vi "_uintGetUintBase.vi"(8 "Error in (no error)":errorcluster, 11 "UintClass in":refnum<class "UintClass.lvclass">) -> (0 "Error out":errorcluster, 1 "Base out":T1=10 caption="Base (decimal)" items=["Binary"=2, "Octal"=8, "Decimal"=10, "Hexadecimal"=16, "Hexatrigesimal"=36, "ASCII"=64], 2 "Uint out":u8[](array[numeric]), 3 "UintClass out":refnum<class "UintClass.lvclass">)   [LabVIEW 2011]
uses:
  UintClass.lvclass
  enumBase.ctl
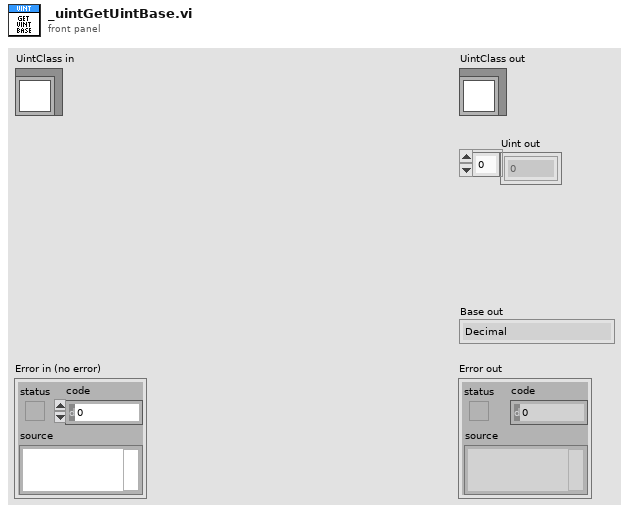
[diagram p1: front panel]
types:
  T1 = typedef "UintClass.lvclass/enumBase.ctl" = u16
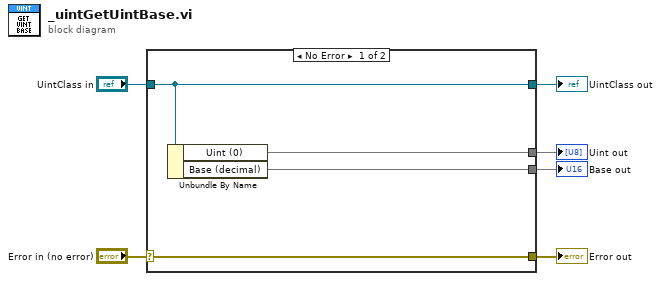
[diagram p0: block diagram]
diagram:
  n1 = case shown="No Error" "Error in (no error)" {
    selector: "Error in (no error)" -> [w10 w11]
    tunnel: [w10 w11] -> w5
    tunnel: [w9 w12] -> w3
    tunnel: "UintClass in" -> [w9 w12]
    tunnel: [w8 _] -> w2
    tunnel: [w7 _] -> w1
    frame No Error {
      n2 = Unbundle By Name(w9) -> ("Uint (0)"=w7, "Base (decimal)"=w8)
    }
    frame Error {
    }
  }
  "Error out" <- w5
  "UintClass out" <- w3
  "Base out" <- w2
  "Uint out" <- w1
